vi "Loop_PDP_SEN.vi"() -> ()   [LabVIEW 2017, in "System_Status.lvlib"]
uses:
  System_Status.lvlib
  TypeDef/CLUSTER_PDP_Status.ctl
  TypeDef/CLUSTER_PDP_Faults.ctl
  <vilib>/Rock Robotics/WPI/DriverStation/WPI_DriverStationRobotMode2.ctl
  Globals/Global_STOP.vi
  Robot Global Data.vi
  Global_SEN Write_Data.vi
panel:
  in  "PDP ID":i32
  out "Cycle Time (S)":dbl format="%.3g"
  in  "Target Time(ms)":u32=50
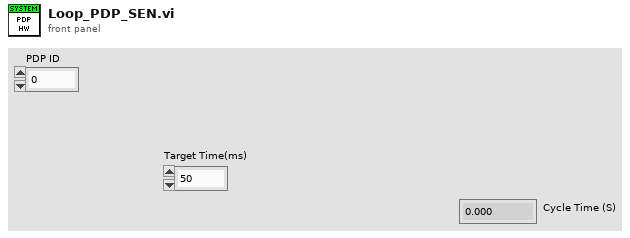
[diagram p1: front panel]
types:
  T1 = typedef "WPI_DriverStationRobotMode2.ctl" = enum16{"Autonomous Disabled", "Autonomous Enabled", "Teleop Disabled", "Teleop Enabled", "Disconnected", "Finish", "Test Disabled", "Test Enabled", "Emergency Stopped"}
  T2 = typedef "CLUSTER_PDP_Status.ctl" = cluster{"PDP Faults":T3, "All Currents (A)":dbl[], "Energy (J)":dbl, "Power (W)":dbl, "Voltage (V)":dbl}
  T3 = typedef "CLUSTER_PDP_Faults.ctl" = cluster{"Current Faults":bool[], "Batt V Fault":bool, "Temp Fault":bool, "HW Fault":bool}
  T4 = cluster{"PDP ID":i32, "Target Time(ms)":u32, "Current Time":timestamp, "Previous Time":timestamp, "Cycle Time (S)":dbl, "PDP Status":T2, "Robot Mode":T1}
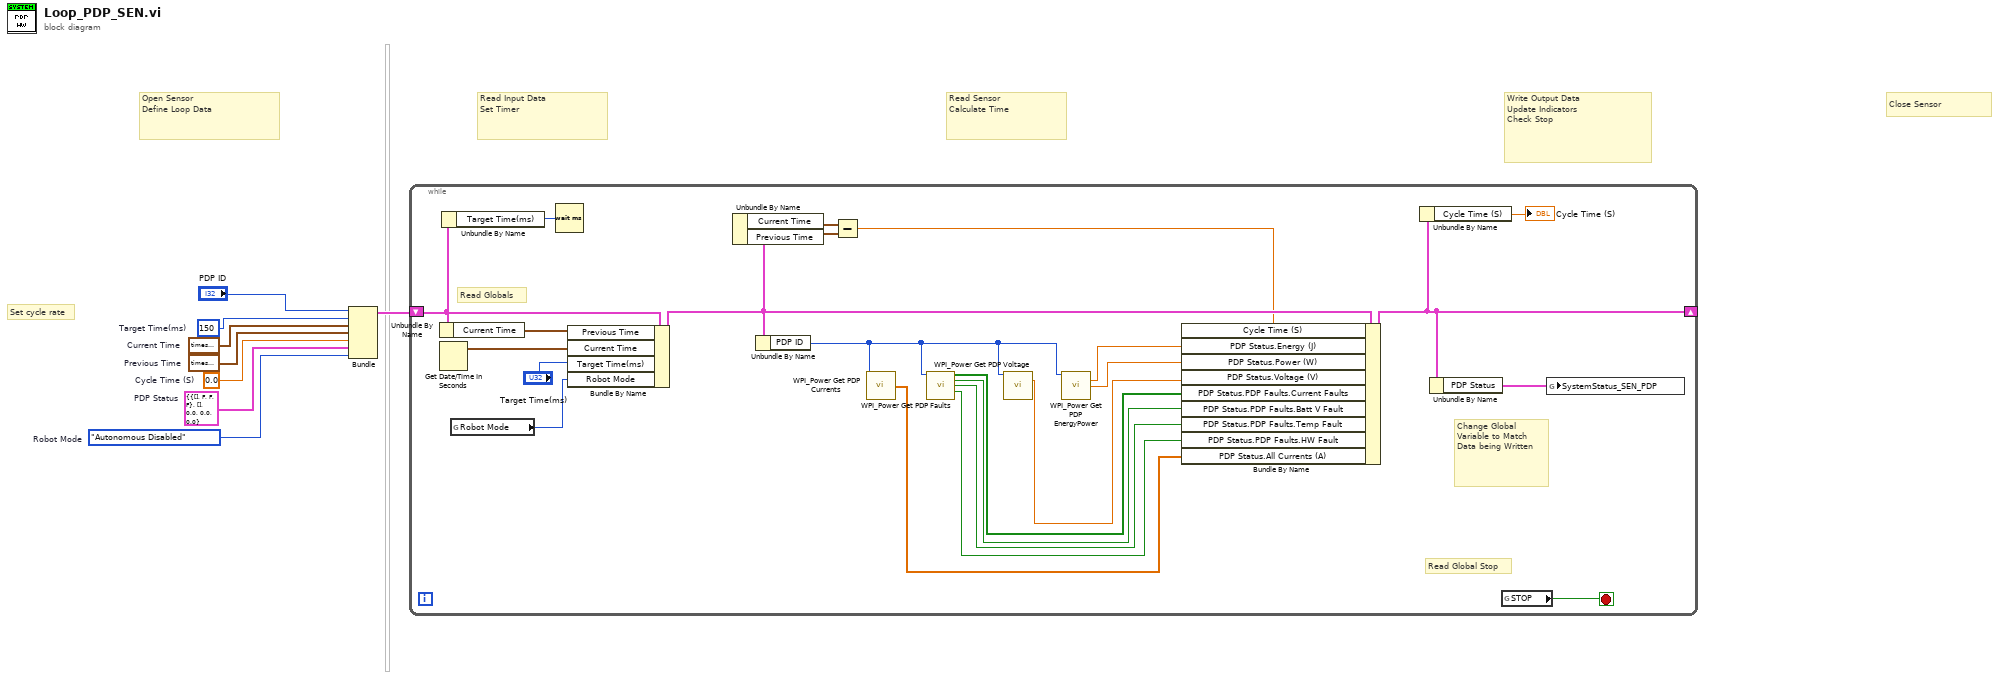
[diagram p0: block diagram]
diagram:
  w1 = WPI_DriverStationRobotMode2."Autonomous Disabled"  # Robot Mode
  w2 = T2 {"PDP Faults"={"Current Faults"=[], "Batt V Fault"=FALSE, "Temp Fault"=FALSE, "HW Fault"=FALSE}, "All Currents (A)"=[], "Energy (J)"=0.0, "Power (W)"=0.0, "Voltage (V)"=0.0}  # PDP Status
  w4 = 0.0  # Cycle Time (S)
  w8 = timestamp(0 s since 1904-01-01)  # Previous Time
  w7 = timestamp(0 s since 1904-01-01)  # Current Time
  w6 = u32 150  # Target Time(ms)
  # "Close Sensor"
  # "Write Output Data\nUpdate Indicators\nCheck Stop"
  # "Read Sensor\nCalculate Time"
  # "Read Input Data\nSet Timer"
  # "Open Sensor\nDefine Loop Data"
  # "Set cycle rate"
  n1 = Bundle("PDP ID"="PDP ID", "Target Time(ms)"=w6, "Current Time"=w7, "Previous Time"=w8, "Cycle Time (S)"=w4, "PDP Status"=w2, "Robot Mode"=w1) -> (w5:T4)  [unwired: 1 in]
  n2 = while {
    shift-right: [w21] -> _
    shift-left: w5 -> [w23]
    stop <- w31 stop-if-true
    # "Change Global\nVariable to Match\nData being Written"
    # "Read Globals"
    # "Read Global Stop"
    n3 = Unbundle By Name(w23) -> ("Current Time"=w28:timestamp)
    n4 = Get Date/Time In Seconds() -> (seconds since 1Jan1904=w29:timestamp)
    n5 = Unbundle By Name(w23) -> ("Target Time(ms)"=w22:u32)
    n6 = global read "Robot Global Data.vi" "Robot Mode"() -> (w9:T1)
    n7 = Wait (ms)(milliseconds to wait=w22) -> ()  [unwired: 1 out]
    n8 = Bundle By Name(cluster=w23, "Previous Time"=w28, "Current Time"=w29, "Target Time(ms)"="Target Time(ms)", "Robot Mode"=w9) -> (w24:T4)
    n9 = Unbundle By Name(w24) -> ("Current Time"=w27:timestamp, "Previous Time"=w26:timestamp)
    n10 = Unbundle By Name(w24) -> ("PDP ID"=w18:i32)
    n11 = Subtract(x=w27, y=w26) -> (x-y=w19:dbl)
    n12 = call <vilib>:"WPI_Power Get PDP Currents.vi"("Power Distribution Panel (0)"=w18) -> ("all currents (A)"=w17:dbl[])  [unwired: 12 in, 2 out]
    n13 = call <vilib>:"WPI_Power Get PDP Faults.vi"("Power Distribution Panel (0)"=w18) -> ("Current Faults"=w16:bool[], "Battery Voltage Fault"=w15:bool, "Temperature Fault"=w14:bool, "Hardware Fault"=w13:bool)  [unwired: 10 in, 1 out]
    n14 = call <vilib>:"WPI_Power Get PDP Voltage.vi"("Power Distribution Panel (0)"=w18) -> ("voltage (V)"=w12:dbl)  [unwired: 13 in, 1 out]
    n15 = call <vilib>:"WPI_Power Get PDP EnergyPower.vi"("Power Distribution Panel (0)"=w18) -> ("Energy (J)"=w10:dbl, "Power (W)"=w11:dbl)  [unwired: 12 in, 1 out]
    n16 = Bundle By Name(cluster=w24, "Cycle Time (S)"=w19, "PDP Status.Energy (J)"=w10, "PDP Status.Power (W)"=w11, "PDP Status.Voltage (V)"=w12, "PDP Status.PDP Faults.Current Faults"=w16, "PDP Status.PDP Faults.Batt V Fault"=w15, "PDP Status.PDP Faults.Temp Fault"=w14, "PDP Status.PDP Faults.HW Fault"=w13, "PDP Status.All Currents (A)"=w17) -> (w21:T4)
    n17 = Unbundle By Name(w21) -> ("Cycle Time (S)"=→"Cycle Time (S)":dbl)
    n18 = Unbundle By Name(w21) -> ("PDP Status"=w30:T2)
    n19 = global read "Global_STOP.vi" "STOP"() -> (w31:bool)
    n20 = global write "Global_SEN Write_Data.vi" "SystemStatus_SEN_PDP"(w30) -> ()
  }
